vi "Voltage _AI- Continuous Input.vi"(2 "Stop":bool, 6 "Logging Mode":i32(ring)=10231 items=["Off"=10231, "Log and Read"=15842], 8 "Number of Samples":i32=100, 9 "Sample Rate":dbl=1000.0, 10 "Terminal Configuration":i32(ring)=-1 items=["default"=-1, "RSE"=10083, "NRSE"=10078, "Differential"=10106, "Pseudodifferential"=12529], 11 "Physical Channel":tag="Dev1/ai0") -> (3 "Waveform Graph":waveform(dbl)[](graph))   [LabVIEW 2012]
doc: "This example demonstrates how to continuously acquire buffered voltage measurements using a DAQmx device.\n\nFor instructions on how to connect your signals to the DAQ device, refer to your device documentation."
uses:
  <vilib>/Utility/error.llb/DialogType.ctl
  <vilib>/DAQmx/read.llb/DAQmx Read (Analog 1D Wfm NChan NSamp).vi
  <vilib>/DAQmx/create/channels.llb/DAQmx Create Channel (AI-Voltage-Basic).vi
  <vilib>/DAQmx/configure/timing.llb/DAQmx Timing (Sample Clock).vi
  <vilib>/DAQmx/configure/task.llb/DAQmx Configure Logging (TDMS).vi
  <vilib>/DAQmx/configure/trigger.llb/DAQmx Start Trigger (Digital Edge).vi
  <vilib>/DAQmx/configure/trigger.llb/DAQmx Start Trigger (Analog Edge).vi
  <vilib>/DAQmx/miscellaneous.llb/DAQmx Fill In Error Info.vi
  <resource>/objmgr/daqmx.rc
panel:
  in  "Trigger Type":T1(tab)
  in  "Edge":i32(ring)=10280 items=["Rising"=10280, "Falling"=10171]
  in  "Digital Trigger Source":tag
  in  "Level (V)":dbl format="%0.2f"
  in  "Hysteresis (V)":dbl
  in  "Slope":i32(ring)=10280 items=["Rising"=10280, "Falling"=10171]
  in  "Analog Trigger Source":string="APFI0"
  in  "TDMS File Path":path
  in  "Sample Clock Source":tag="OnboardClock"
  in  "Max Voltage":dbl=10.0
  in  "Min Voltage":dbl=-10.0
  out "Actual Sample Rate":dbl=1000.0 format="%0.2f"
  # "Channel Settings"
  # "Acquired Data"
  # "Timing Settings"
  # "Trigger Settings"
  # "Logging Settings"
  # "To configure and use a start trigger you must have the necessary tab selected above.  Not all hardware supports triggering--refer to your device documentation for more info."
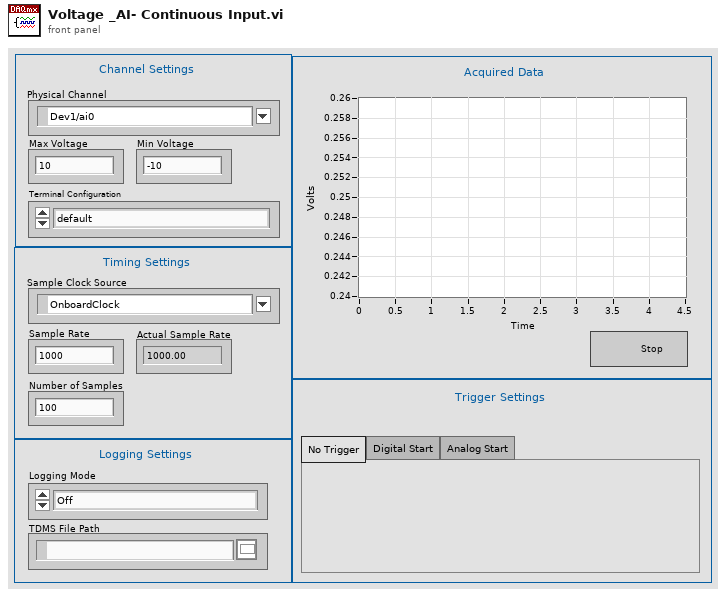
[diagram p1: front panel]
types:
  T1 = enum32{"No Trigger", "Digital Start", "Analog Start"}
  T2 = typedef "DialogType.ctl" = u16
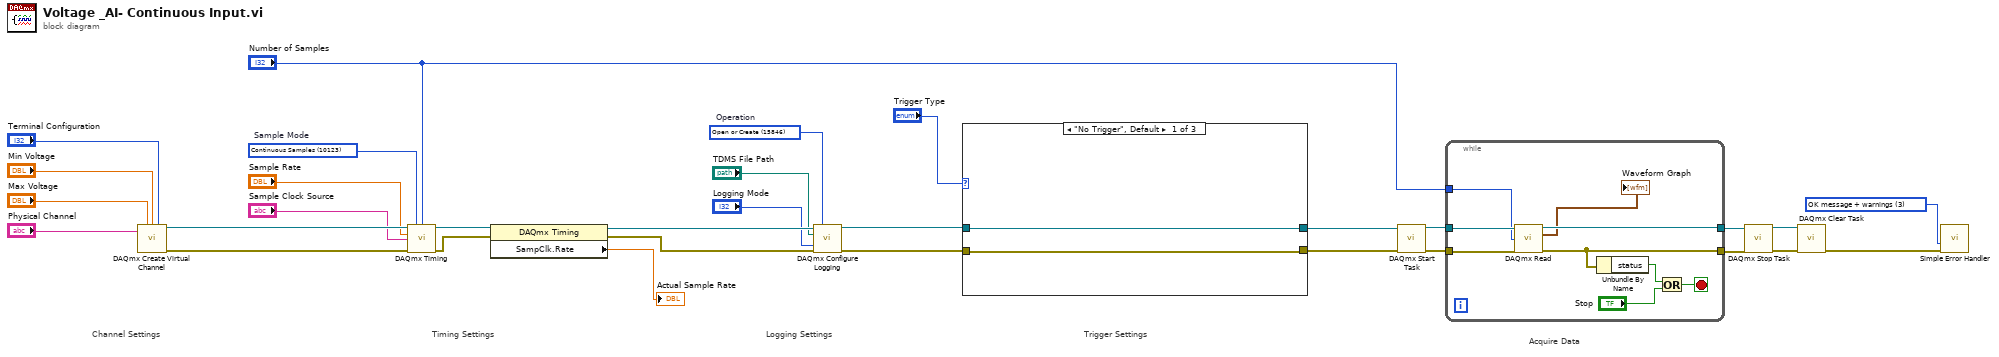
[diagram p0: block diagram]
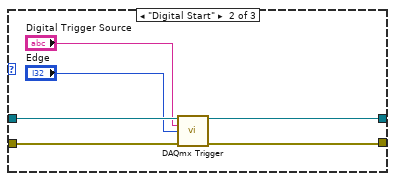
[diagram p2: hidden frame]
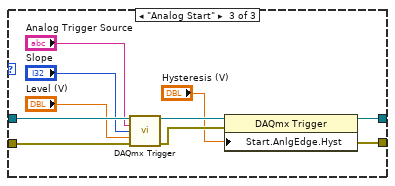
[diagram p3: hidden frame]
diagram:
  w1 = T2 3 items=["no dialog", "OK message", "continue or stop message", "OK message + warnings", "continue/stop + warnings"] ("type of dialog (OK msg:1)")
  w24 = 15846 items=["Open"=10437, "Open or Create"=15846, "Create or Replace"=15847, "Create"=15848]  # Operation
  w29 = 10123 items=["Finite Samples"=10178, "Continuous Samples"=10123, "Hardware Timed Single Point"=12522]  # Sample Mode
  # "Acquire Data"
  # "Trigger Settings"
  # "Timing Settings"
  # "Channel Settings"
  # "Logging Settings"
  n1 = call-poly <vilib>:"DAQmx Create Virtual Channel.vi"("maximum value"="Max Voltage", "minimum value"="Min Voltage", "input terminal configuration"="Terminal Configuration", "physical channels"="Physical Channel") -> ("task out"=w27:refnum<k21>, "error out"=w28:errorcluster)  [unwired: 10 in]
  n2 = call-poly <vilib>:"DAQmx Timing.vi"("task/channels in"=w27, "sample mode"=w29, "samples per channel"="Number of Samples", "rate"="Sample Rate", "source"="Sample Clock Source", "error in"=w28) -> ("task out"=w31:refnum<k21>, "error out"=w30:errorcluster)  [unwired: 8 in]
  n3 = property class="DAQmx Timing"(reference=w31, error in=w30) -> (reference out=w26:refnum<k21>, error out=w25:errorcluster, "SampClk.Rate"=→"Actual Sample Rate":dbl)
  n4 = call-poly <vilib>:"DAQmx Configure Logging.vi"("task/channels in"=w26, "operation"=w24, "file path"="TDMS File Path", "logging mode"="Logging Mode", "error in"=w25) -> ("task out"=w23:refnum<k21>, "error out"=w22:errorcluster)  [unwired: 9 in]
  n5 = case shown="\"No Trigger\", Default" "Trigger Type" {
    tunnel: w23 -> [w33 w39 w49]
    tunnel: w22 -> [w32 w38 w48]
    tunnel: [w33 w37 w46] -> w21
    tunnel: [w32 w36 w45] -> w20
    frame "No Trigger", Default {
    }
    frame "Digital Start" {
      n6 = call-poly <vilib>:"DAQmx Trigger.vi"("task/channels in"=w39, "source"="Digital Trigger Source", "edge"="Edge", "error in"=w38) -> ("task out"=w37:refnum<k21>, "error out"=w36:errorcluster)  [unwired: 10 in]
    }
    frame "Analog Start" {
      n7 = call-poly <vilib>:"DAQmx Trigger.vi"("task/channels in"=w49, "source"="Analog Trigger Source", "slope"="Slope", "level"="Level (V)", "error in"=w48) -> ("task out"=w44:refnum<k21>, "error out"=w43:errorcluster)  [unwired: 9 in]
      n8 = property class="DAQmx Trigger"(reference=w44, error in=w43, "Start.AnlgEdge.Hyst"="Hysteresis (V)") -> (reference out=w46:refnum<k21>, error out=w45:errorcluster)
    }
  }
  n9 = call <vilib>:"DAQmx Start Task.vi"("task/channels in"=w21, "error in"=w20) -> ("task out"=w19:refnum<k21>, "error out"=w18:errorcluster)  [unwired: 12 in]
  n10 = while {
    tunnel: w19 -> [w58]
    tunnel: w18 -> [w57]
    tunnel: [w56] -> w5
    tunnel: [w53] -> w4
    tunnel: "Number of Samples" -> [w50]
    stop <- w51 stop-if-true
    n11 = call-poly <vilib>:"DAQmx Read.vi"("task/channels in"=w58, "number of samples per channel"=w50, "error in"=w57) -> ("task out"=w56:refnum<k21>, "data"=→"Waveform Graph":waveform(dbl)[], "error out"=w53:errorcluster)  [unwired: 10 in]
    n12 = Unbundle By Name(w53) -> ("status"=w52:bool)
    n13 = Or(x=w52, y="Stop") -> (x .or. y?=w51:bool)
  }
  n14 = call <vilib>:"DAQmx Stop Task.vi"("task/channels in"=w5, "error in"=w4) -> ("task out"=w2:refnum<k21>, "error out"=w3:errorcluster)  [unwired: 12 in]
  n15 = call <vilib>:"DAQmx Clear Task.vi"("task in"=w2, "error in"=w3) -> ("error out"=w17:errorcluster)  [unwired: 13 in]
  n16 = call <vilib>:"Simple Error Handler.vi"("type of dialog (OK msg:1)"=w1, "error in (no error)"=w17) -> ()  [unwired: 3 in, 5 out]
